vi "App Run.vi"(8 "error in (no error)":errorcluster, 10 "Core APIs":T3, 11 "DemoApp in":refnum<class "DemoApp.lvclass">) -> (0 "error out":errorcluster)   [LabVIEW 2020, in "VolatusDemo.lvlib" / "DemoApp.lvclass"]
uses:
  DemoApp.lvclass
  Volatus/Core APIs.ctl
  Volatus/VolatusAPI/VolatusAPI.lvclass
  Volatus/Event API/EventAPI.lvclass
  Volatus/Event.ctl
  Volatus/Event Level.ctl
  DemoApp.lvclass/DemoApp.ctl
  ChartGuiTask/ChartGuiTask.lvclass
  C:/dev/lv20CE/relink/lv-volatus/Volatus/Task/Task.lvclass
  SimTask/SimTask.lvclass
  Volatus/Volatus.lvlib
  Volatus/TelemetryAPI/TelemetryAPI.lvclass
panel:
  out "Events":T1[](array[typedef])
  in  "Add Sim":bool
  in  "Add Chart":bool
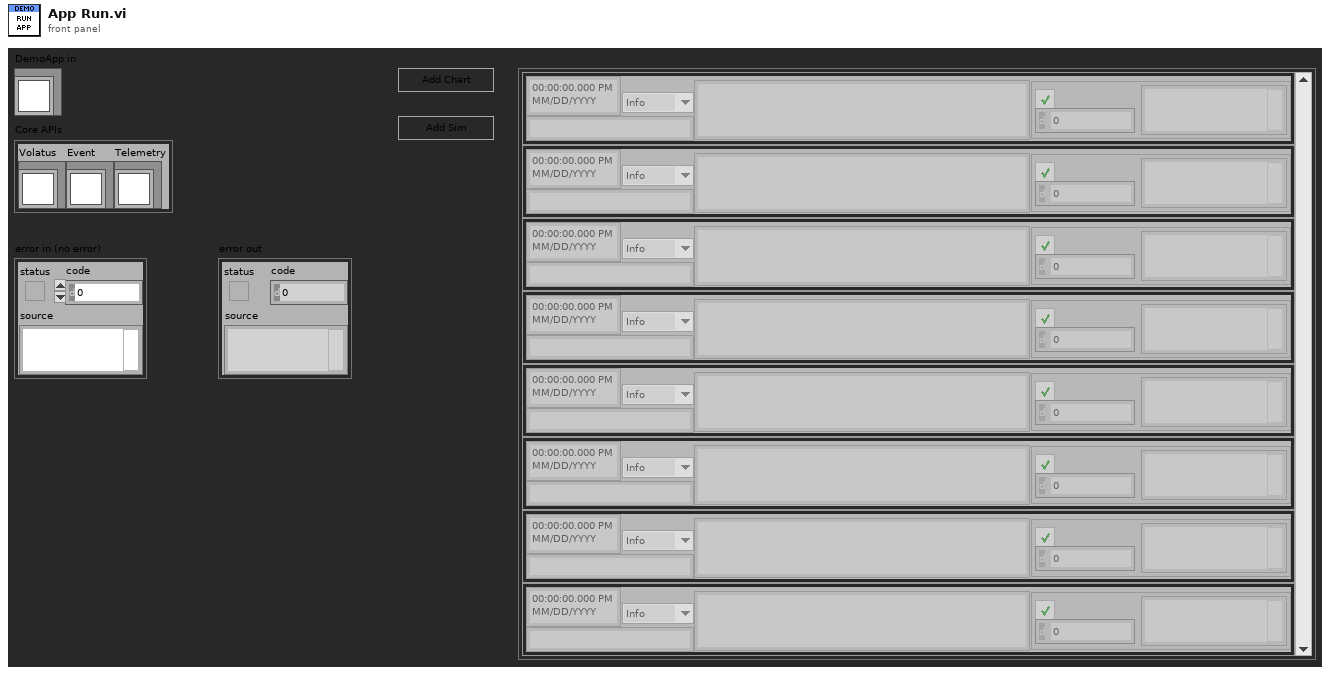
[diagram p1: front panel]
types:
  T1 = typedef "Volatus.lvlib/Event.ctl" = cluster{"Level":T2, "Context":string, "Message":string, "Error":errorcluster, "Time Stamp":timestamp}
  T2 = typedef "Volatus.lvlib/Event Level.ctl" = enum16{"Debug", "Info", "Warning", "Error"}
  T3 = typedef "Volatus.lvlib/Core APIs.ctl" = cluster{"Volatus":refnum<class "VolatusAPI.lvclass">, "Event":refnum<class "EventAPI.lvclass">, "Telemetry":refnum<class "TelemetryAPI.lvclass">}
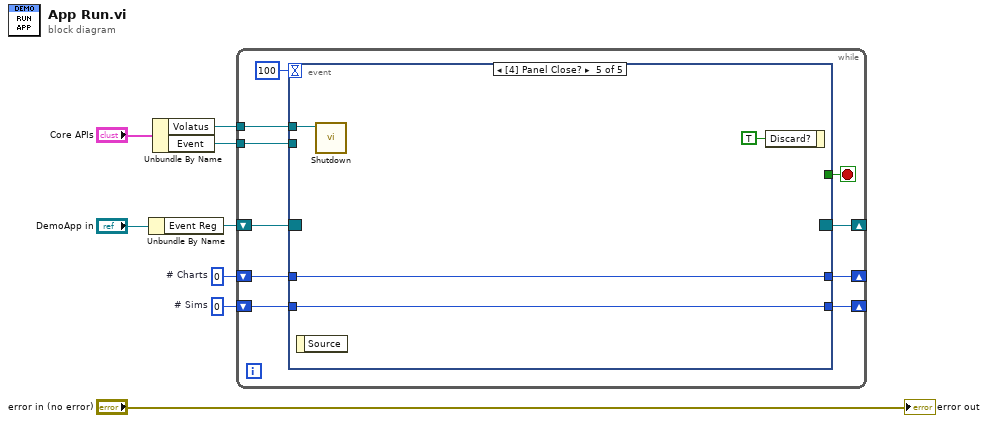
[diagram p0: block diagram]
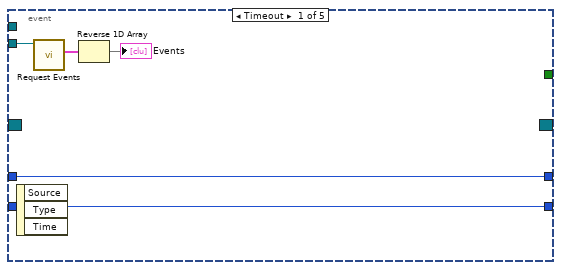
[diagram p2: hidden frame]
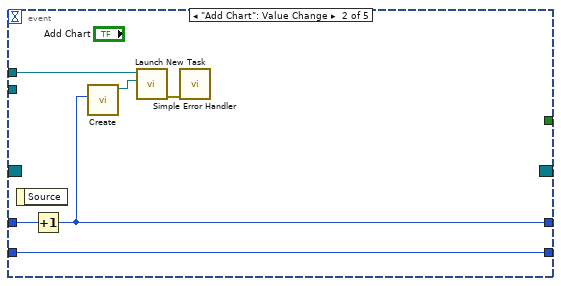
[diagram p3: hidden frame]
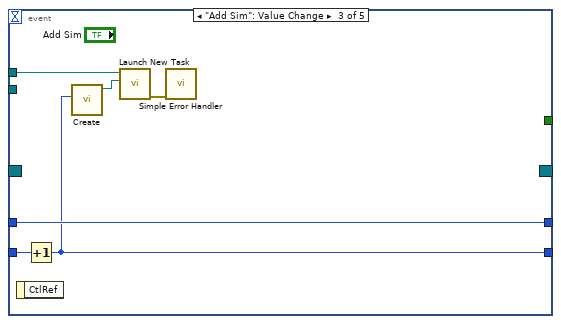
[diagram p4: hidden frame]
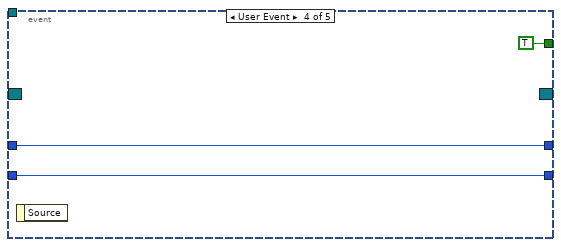
[diagram p5: hidden frame]
diagram:
  w1 = 0  # # Sims
  w2 = 0  # # Charts
  n1 = Unbundle By Name("DemoApp in") -> ("Event Reg"=w7:refnum<event-registration>)
  n2 = Unbundle By Name("Core APIs") -> ("Volatus"=w4:refnum<class "VolatusAPI.lvclass">, "Event"=w5:refnum<class "EventAPI.lvclass">)
  n3 = while {
    shift-right: [w15] -> _
    shift-left: w7 -> [w16]
    tunnel: w5 -> [w17]
    tunnel: w4 -> [w14]
    shift-right: [w12] -> _
    shift-left: w2 -> [w13]
    shift-right: [w10] -> _
    shift-left: w1 -> [w11]
    stop <- w9 stop-if-true
    n4 = event shown="[4] Panel Close?" {
      selector: w16 -> [_ _ _ _ _]
      dyn-events: [_ _ _ _ _] -> w15
      timeout: 100 -> [_ _ _ _ _]
      tunnel: w17 -> [w23 _ _ _ _]
      tunnel: w14 -> [_ w29 w32 _ w39]
      tunnel: w13 -> [w20 w27 w35 w38 w42]
      tunnel: [w20 w24 w35 w38 w42] -> w12
      tunnel: w11 -> [w19 w26 w34 w37 w41]
      tunnel: [w19 w26 w33 w37 w41] -> w10
      tunnel: [_ _ _ TRUE _] -> w9
      event Timeout {
        n5 = event-data() -> ()  [unwired: 1 in, 3 out]
        n6 = call "Request Events.vi"("EventAPI in"=w23) -> ("Events"=w22:T1[])  [unwired: 8 in, 2 out]
        n7 = Reverse 1D Array(array=w22) -> (reversed array=→"Events":T1[])
      }
      event "Add Chart": Value Change {
        n8 = event-data() -> ()  [unwired: 1 in, 1 out]
        n9 = Increment(x=w27) -> (x+1=w24:i32)
        n10 = call "Create.vi"("Number"=w24) -> ("ChartGuiTask out"=w25:refnum<class "ChartGuiTask.lvclass">)  [unwired: 9 in, 1 out]
        n11 = call "Launch New Task.vi"("Task"=w25, "VolatusAPI in"=w29) -> ("error out"=w28:errorcluster)  [unwired: 8 in, 1 out]
        n12 = call <vilib>:"Simple Error Handler.vi"("error in (no error)"=w28) -> ()  [unwired: 4 in, 5 out]
      }
      event "Add Sim": Value Change {
        n13 = event-data() -> ()  [unwired: 1 in, 1 out]
        n14 = Increment(x=w34) -> (x+1=w33:i32)
        n15 = call "Create.vi"("Number"=w33) -> ("SimTask out"=w31:refnum<class "SimTask.lvclass">)  [unwired: 9 in, 1 out]
        n16 = call "Launch New Task.vi"("Task"=w31, "VolatusAPI in"=w32) -> ("error out"=w30:errorcluster)  [unwired: 8 in, 1 out]
        n17 = call <vilib>:"Simple Error Handler.vi"("error in (no error)"=w30) -> ()  [unwired: 4 in, 5 out]
      }
      event User Event {
        n18 = event-data() -> ()  [unwired: 1 in, 1 out]
      }
      event Panel Close? {
        n19 = event-data() -> ()  [unwired: 1 in, 1 out]
        n20 = call "Shutdown.vi"("VolatusAPI in"=w39) -> ()  [unwired: 9 in, 2 out]
        n21 = event-data("Discard?"=TRUE) -> ()  [unwired: 1 in, 1 out]
      }
    }
  }
  "error out" <- "error in (no error)"
